vi "Desonatter Torque data read.vi"() -> (3 "Result":bool, 10 "Parameter":u8, 11 "Channel":i32)   [LabVIEW 2015]
uses:
  Galobal variable_TI.vi
  Project Setup/Globle Variable/GR_Servo.vi
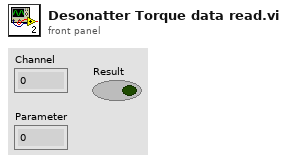
[diagram p1: front panel]
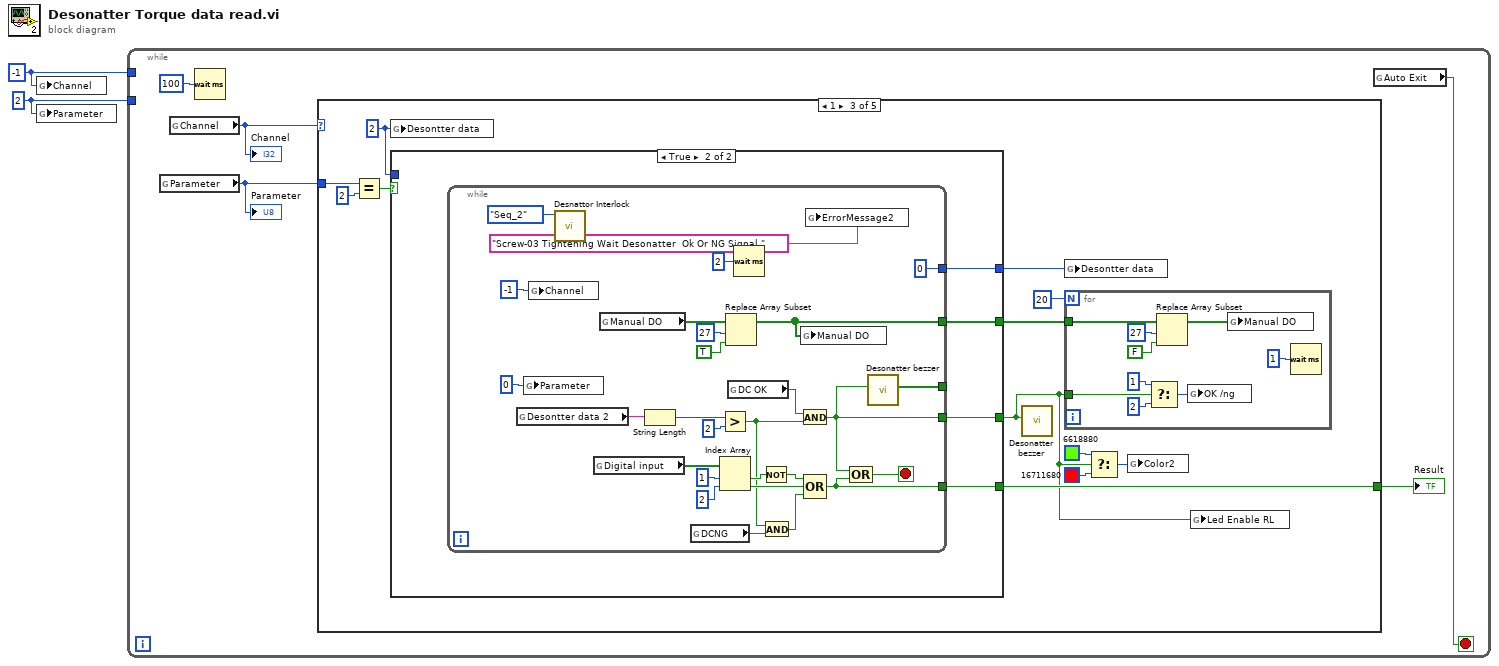
[diagram p0: block diagram]
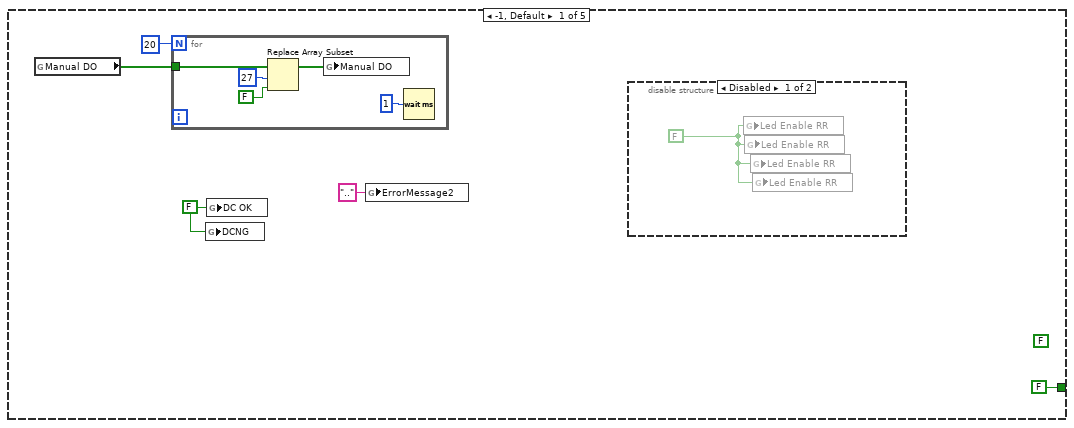
[diagram p2: hidden frame]
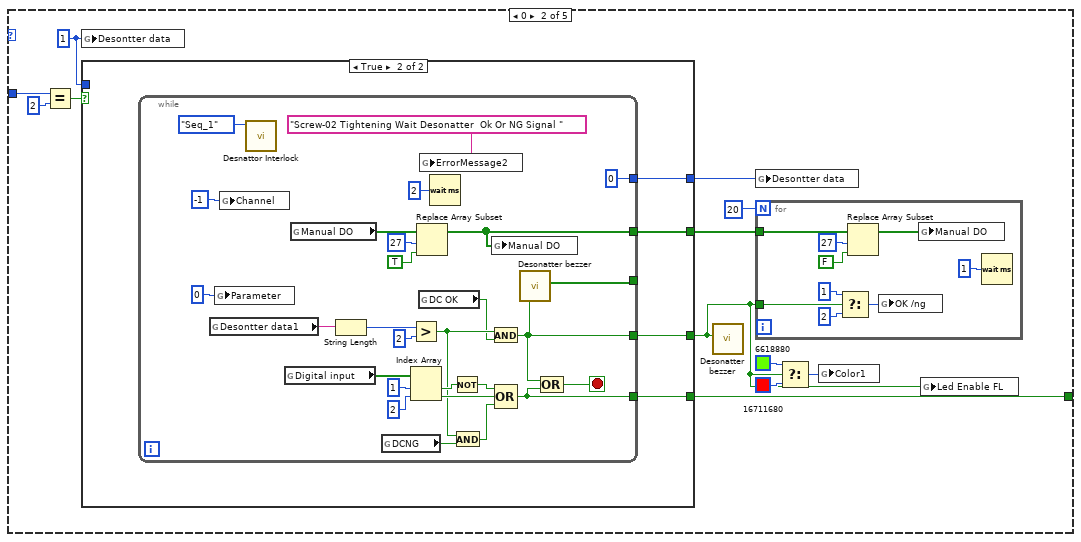
[diagram p4: hidden frame]
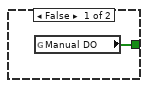
[diagram p5: hidden frame]
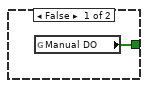
[diagram p6: hidden frame]
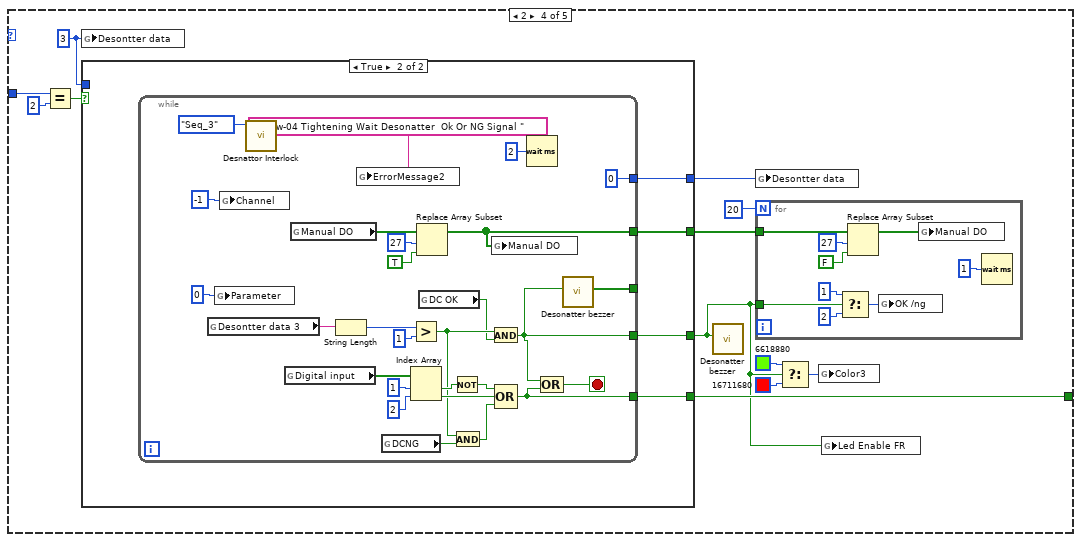
[diagram p7: hidden frame]
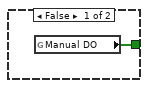
[diagram p8: hidden frame]
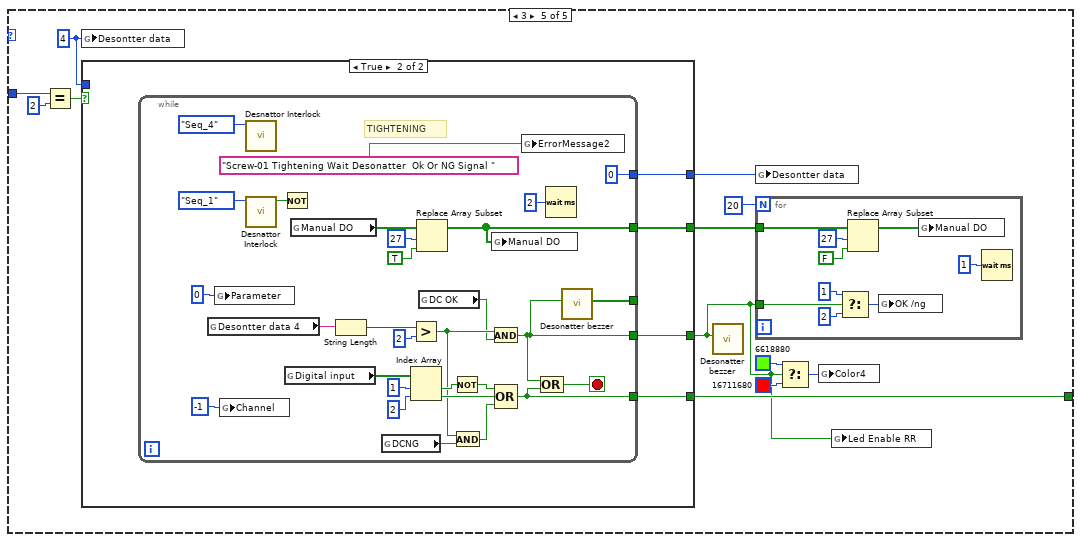
[diagram p9: hidden frame]
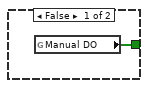
[diagram p10: hidden frame]
diagram:
  w1 = u8 2 ("Parameter")
  w2 = -1 ("Channel")
  n1 = global write "Galobal variable_TI.vi" "Channel"(w2) -> ()
  n2 = global write "Galobal variable_TI.vi" "Parameter"(w1) -> ()
  n3 = while {
    tunnel: w2 -> [_]
    tunnel: w1 -> [_]
    stop <- w6 stop-if-true
    n4 = global read "Galobal variable_TI.vi" "Parameter"() -> (w4:u8)
    "Parameter" <- w4
    n5 = global read "Galobal variable_TI.vi" "Channel"() -> (w5:i32)
    "Channel" <- w5
    n6 = Wait (ms)(milliseconds to wait=u32 100) -> ()  [unwired: 1 out]
    n7 = case shown="1" w5 {
      tunnel: w4 -> [_ w30 w83 w134 w187]
      tunnel: [FALSE w27 w82 w133 w186] -> w7
      frame -1, Default {
        (unwired) FALSE
        w8 = FALSE ("DC OK")
        n8 = global read "Galobal variable_TI.vi" "Manual DO"() -> (w11:bool[])
        n9 = for {
          N: 20 -> [_]
          tunnel: w11 -> [w18]
          n10 = Replace Array Subset(array=w18, new element=FALSE ("new element/subarray"), index=27) -> (w17:bool[])
          n11 = global write "Galobal variable_TI.vi" "Manual DO"(w17) -> ()
          n12 = Wait (ms)(milliseconds to wait=u32 1) -> ()  [unwired: 1 out]
        }
        n13 = global write "Galobal variable_TI.vi" "DCNG"(w8) -> ()
        n14 = global write "Galobal variable_TI.vi" "DC OK"(w8) -> ()
        n15 = global write "GR_Servo.vi" "ErrorMessage2"(".." ("ErrorMessage2")) -> ()
        n16 = disable-structure shown="Disabled" {
          frame Disabled {
            w13 = FALSE
            n17 = global write "Galobal variable_TI.vi" "Led Enable RR"(w13) -> ()
            n18 = global write "Galobal variable_TI.vi" "Led Enable RR"(w13) -> ()
            n19 = global write "Galobal variable_TI.vi" "Led Enable RR"(w13) -> ()
            n20 = global write "Galobal variable_TI.vi" "Led Enable RR"(w13) -> ()
          }
          frame Enabled {
          }
        }
      }
      frame 0 {
        w22 = 1 ("Desontter data")
        n21 = Equal?(x=w30, y=u8 2) -> (x = y?=w28:bool)
        n22 = global write "Galobal variable_TI.vi" "Desontter data"(w22) -> ()
        n23 = case shown="True" w28 {
          tunnel: [_ w44] -> w27
          tunnel: [_ w43] -> w26
          tunnel: [_ w42] -> w19
          tunnel: w22 -> [_ _]
          tunnel: [w40 w41] -> w21
          frame False {
            n24 = global read "Galobal variable_TI.vi" "Manual DO"() -> (w40:bool[])
          }
          frame True {
            n25 = while {
              tunnel: [w63] -> w44
              tunnel: [0 ("y")] -> w43
              tunnel: [w45] -> w42
              tunnel: [w53] -> w41
              tunnel: [w48] -> _
              stop <- w62 stop-if-true
              n26 = global read "Galobal variable_TI.vi" "Desontter data1"() -> (w66:string)
              n27 = global write "Galobal variable_TI.vi" "Parameter"(u8 0 ("Parameter")) -> ()
              n28 = global write "Galobal variable_TI.vi" "Channel"(-1 ("Channel")) -> ()
              n29 = call "Desnattor Interlock.vi"("Seq1"=enum16{"Seq_1", "Seq_2", "Seq_3", "Seq_4"}."Seq_1") -> ()  [unwired: 10 in, 1 out]
              n30 = global read "Galobal variable_TI.vi" "Digital input"() -> (w60:bool[])
              n31 = global read "Galobal variable_TI.vi" "Manual DO"() -> (w55:bool[])
              n32 = String Length(string=w66) -> (length=w65:i32)
              n33 = global read "Galobal variable_TI.vi" "DCNG"() -> (w58:bool)
              n34 = Greater?(x=w65, y=2) -> (0:w59:bool)
              n35 = Index Array(array=w60, index #1=1 ("index"), index #2=2 ("index")) -> (element #1=w69:bool, element #2=w67:bool)
              n36 = Replace Array Subset(array=w55, new element=TRUE ("new element/subarray"), index=27) -> (w53:bool[])
              n37 = global read "Galobal variable_TI.vi" "DC OK"() -> (w49:bool)
              n38 = global write "GR_Servo.vi" "ErrorMessage2"("Screw-02 Tightening Wait Desonatter  Ok Or NG Signal ") -> ()
              n39 = Wait (ms)(milliseconds to wait=u32 2) -> ()  [unwired: 1 out]
              n40 = Not(x=w69) -> (.not. x?=w68:bool)
              n41 = And(x=w59, y=w58) -> (x .and. y?=w57:bool)
              n42 = And(x=w59, y=w49) -> (x .and. y?=w45:bool)
              n43 = global write "Galobal variable_TI.vi" "Manual DO"(w53) -> ()
              n44 = Compound Arithmetic op=OR(w68, w67, w57) -> (w63:bool)
              n45 = call "Desonatter bezzer.vi"("OK"=w45) -> ("Array"=w48:bool[])  [unwired: 10 in]
              n46 = Compound Arithmetic op=OR(w45, w63) -> (w62:bool)
            }
          }
        }
        n47 = call "Desonatter bezzer.vi"("OK"=w19) -> ()  [unwired: 10 in, 1 out]
        n48 = global write "Galobal variable_TI.vi" "Desontter data"(w26) -> ()
        n49 = for {
          N: 20 -> [_]
          tunnel: w21 -> [w39]
          tunnel: w19 -> [w31]
          n50 = Select(t=1, s=w31, f=2) -> (s? t:f=w34:i32)
          n51 = Replace Array Subset(array=w39, new element=FALSE ("new element/subarray"), index=27) -> (w38:bool[])
          n52 = global write "Galobal variable_TI.vi" "OK /ng"(w34) -> ()
          n53 = global write "Galobal variable_TI.vi" "Manual DO"(w38) -> ()
          n54 = Wait (ms)(milliseconds to wait=u32 1) -> ()  [unwired: 1 out]
        }
        n55 = Select(t=u32 6618880 ("Color Box"), s=w19, f=u32 16711680 ("Color Box")) -> (s? t:f=w23:u32)
        n56 = global write "Galobal variable_TI.vi" "Color1"(w23) -> ()
        n57 = global write "Galobal variable_TI.vi" "Led Enable FL"(w19) -> ()
      }
      frame 1 {
        w75 = 2 ("Desontter data")
        n58 = Equal?(x=w83, y=u8 2) -> (x = y?=w80:bool)
        n59 = global write "Galobal variable_TI.vi" "Desontter data"(w75) -> ()
        n60 = case shown="True" w80 {
          tunnel: [_ w97] -> w82
          tunnel: [_ w96] -> w79
          tunnel: [_ w95] -> w72
          tunnel: w75 -> [_ _]
          tunnel: [w93 w94] -> w73
          frame False {
            n61 = global read "Galobal variable_TI.vi" "Manual DO"() -> (w93:bool[])
          }
          frame True {
            n62 = while {
              tunnel: [w115] -> w97
              tunnel: [0 ("y")] -> w96
              tunnel: [w98] -> w95
              tunnel: [w105] -> w94
              tunnel: [w101] -> _
              stop <- w114 stop-if-true
              n63 = global read "Galobal variable_TI.vi" "Desontter data 2"() -> (w118:string)
              n64 = global write "Galobal variable_TI.vi" "Parameter"(u8 0 ("Parameter")) -> ()
              n65 = global write "Galobal variable_TI.vi" "Channel"(-1 ("Channel")) -> ()
              n66 = call "Desnattor Interlock.vi"("Seq1"=enum16{"Seq_1", "Seq_2", "Seq_3", "Seq_4"}."Seq_2") -> ()  [unwired: 10 in, 1 out]
              n67 = global read "Galobal variable_TI.vi" "Digital input"() -> (w124:bool[])
              n68 = global read "Galobal variable_TI.vi" "Manual DO"() -> (w108:bool[])
              n69 = String Length(string=w118) -> (length=w117:i32)
              n70 = global read "Galobal variable_TI.vi" "DCNG"() -> (w111:bool)
              n71 = Greater?(x=w117, y=2) -> (0:w112:bool)
              n72 = Index Array(array=w124, index #1=1 ("index"), index #2=2 ("index")) -> (element #1=w121:bool, element #2=w119:bool)
              n73 = Replace Array Subset(array=w108, new element=TRUE ("new element/subarray"), index=27) -> (w105:bool[])
              n74 = global read "Galobal variable_TI.vi" "DC OK"() -> (w102:bool)
              n75 = Wait (ms)(milliseconds to wait=u32 2) -> ()  [unwired: 1 out]
              n76 = Not(x=w121) -> (.not. x?=w120:bool)
              n77 = And(x=w112, y=w111) -> (x .and. y?=w110:bool)
              n78 = And(x=w102, y=w112) -> (x .and. y?=w98:bool)
              n79 = global write "Galobal variable_TI.vi" "Manual DO"(w105) -> ()
              n80 = Compound Arithmetic op=OR(w120, w119, w110) -> (w115:bool)
              n81 = global write "GR_Servo.vi" "ErrorMessage2"("Screw-03 Tightening Wait Desonatter  Ok Or NG Signal ") -> ()
              n82 = Compound Arithmetic op=OR(w98, w115) -> (w114:bool)
              n83 = call "Desonatter bezzer.vi"("OK"=w98) -> ("Array"=w101:bool[])  [unwired: 10 in]
            }
          }
        }
        n84 = call "Desonatter bezzer.vi"("OK"=w72) -> ()  [unwired: 10 in, 1 out]
        n85 = global write "Galobal variable_TI.vi" "Desontter data"(w79) -> ()
        n86 = for {
          N: 20 -> [_]
          tunnel: w73 -> [w92]
          tunnel: w72 -> [w87]
          n87 = Select(t=1, s=w87, f=2) -> (s? t:f=w86:i32)
          n88 = Replace Array Subset(array=w92, new element=FALSE ("new element/subarray"), index=27) -> (w91:bool[])
          n89 = global write "Galobal variable_TI.vi" "OK /ng"(w86) -> ()
          n90 = global write "Galobal variable_TI.vi" "Manual DO"(w91) -> ()
          n91 = Wait (ms)(milliseconds to wait=u32 1) -> ()  [unwired: 1 out]
        }
        n92 = Select(t=u32 6618880 ("Color Box"), s=w72, f=u32 16711680 ("Color Box")) -> (s? t:f=w78:u32)
        n93 = global write "Galobal variable_TI.vi" "Color2"(w78) -> ()
        n94 = global write "Galobal variable_TI.vi" "Led Enable RL"(w72) -> ()
      }
      frame 2 {
        w128 = 3 ("Desontter data")
        n95 = Equal?(x=w134, y=u8 2) -> (x = y?=w135:bool)
        n96 = global write "Galobal variable_TI.vi" "Desontter data"(w128) -> ()
        n97 = case shown="True" w135 {
          tunnel: [_ w150] -> w133
          tunnel: [_ w149] -> w132
          tunnel: [_ w148] -> w125
          tunnel: w128 -> [_ _]
          tunnel: [w146 w147] -> w126
          frame False {
            n98 = global read "Galobal variable_TI.vi" "Manual DO"() -> (w146:bool[])
          }
          frame True {
            n99 = while {
              tunnel: [w168] -> w150
              tunnel: [0 ("y")] -> w149
              tunnel: [w151] -> w148
              tunnel: [w158] -> w147
              tunnel: [w154] -> _
              stop <- w167 stop-if-true
              n100 = global read "Galobal variable_TI.vi" "Desontter data 3"() -> (w171:string)
              n101 = global write "Galobal variable_TI.vi" "Parameter"(u8 0 ("Parameter")) -> ()
              n102 = global write "Galobal variable_TI.vi" "Channel"(-1 ("Channel")) -> ()
              n103 = call "Desnattor Interlock.vi"("Seq1"=enum16{"Seq_1", "Seq_2", "Seq_3", "Seq_4"}."Seq_3") -> ()  [unwired: 10 in, 1 out]
              n104 = global read "Galobal variable_TI.vi" "Digital input"() -> (w177:bool[])
              n105 = global read "Galobal variable_TI.vi" "Manual DO"() -> (w161:bool[])
              n106 = String Length(string=w171) -> (length=w170:i32)
              n107 = global write "GR_Servo.vi" "ErrorMessage2"("Screw-04 Tightening Wait Desonatter  Ok Or NG Signal ") -> ()
              n108 = global read "Galobal variable_TI.vi" "DCNG"() -> (w163:bool)
              n109 = Greater?(x=w170, y=1) -> (0:w165:bool)
              n110 = Index Array(array=w177, index #1=1 ("index"), index #2=2 ("index")) -> (element #1=w174:bool, element #2=w172:bool)
              n111 = Replace Array Subset(array=w161, new element=TRUE ("new element/subarray"), index=27) -> (w158:bool[])
              n112 = global read "Galobal variable_TI.vi" "DC OK"() -> (w155:bool)
              n113 = Not(x=w174) -> (.not. x?=w173:bool)
              n114 = And(x=w165, y=w163) -> (x .and. y?=w164:bool)
              n115 = And(x=w165, y=w155) -> (x .and. y?=w151:bool)
              n116 = global write "Galobal variable_TI.vi" "Manual DO"(w158) -> ()
              n117 = Compound Arithmetic op=OR(w173, w172, w164) -> (w168:bool)
              n118 = Wait (ms)(milliseconds to wait=u32 2) -> ()  [unwired: 1 out]
              n119 = Compound Arithmetic op=OR(w151, w168) -> (w167:bool)
              n120 = call "Desonatter bezzer.vi"("OK"=w151) -> ("Array"=w154:bool[])  [unwired: 10 in]
            }
          }
        }
        n121 = call "Desonatter bezzer.vi"("OK"=w125) -> ()  [unwired: 10 in, 1 out]
        n122 = global write "Galobal variable_TI.vi" "Desontter data"(w132) -> ()
        n123 = for {
          N: 20 -> [_]
          tunnel: w126 -> [w145]
          tunnel: w125 -> [w137]
          n124 = Select(t=1, s=w137, f=2) -> (s? t:f=w140:i32)
          n125 = Replace Array Subset(array=w145, new element=FALSE ("new element/subarray"), index=27) -> (w144:bool[])
          n126 = global write "Galobal variable_TI.vi" "OK /ng"(w140) -> ()
          n127 = global write "Galobal variable_TI.vi" "Manual DO"(w144) -> ()
          n128 = Wait (ms)(milliseconds to wait=u32 1) -> ()  [unwired: 1 out]
        }
        n129 = Select(t=u32 6618880 ("Color Box"), s=w125, f=u32 16711680 ("Color Box")) -> (s? t:f=w131:u32)
        n130 = global write "Galobal variable_TI.vi" "Color3"(w131) -> ()
        n131 = global write "Galobal variable_TI.vi" "Led Enable FR"(w125) -> ()
      }
      frame 3 {
        w181 = 4 ("Desontter data")
        n132 = Equal?(x=w187, y=u8 2) -> (x = y?=w188:bool)
        n133 = global write "Galobal variable_TI.vi" "Desontter data"(w181) -> ()
        n134 = case shown="True" w188 {
          tunnel: [_ w203] -> w186
          tunnel: [_ w202] -> w185
          tunnel: [_ w201] -> w178
          tunnel: w181 -> [_ _]
          tunnel: [w199 w200] -> w179
          frame False {
            n135 = global read "Galobal variable_TI.vi" "Manual DO"() -> (w199:bool[])
          }
          frame True {
            n136 = while {
              tunnel: [w223] -> w203
              tunnel: [0 ("Desontter data")] -> w202
              tunnel: [w204] -> w201
              tunnel: [w210] -> w200
              tunnel: [w206] -> _
              stop <- w222 stop-if-true
              # "TIGHTENING"
              n137 = global read "Galobal variable_TI.vi" "Desontter data 4"() -> (w226:string)
              n138 = global write "Galobal variable_TI.vi" "Parameter"(u8 0 ("Parameter")) -> ()
              n139 = global write "Galobal variable_TI.vi" "Channel"(-1 ("Channel")) -> ()
              n140 = call "Desnattor Interlock.vi"("Seq1"=enum16{"Seq_1", "Seq_2", "Seq_3", "Seq_4"}."Seq_4") -> ()  [unwired: 10 in, 1 out]
              n141 = call "Desnattor Interlock.vi"("Seq1"=enum16{"Seq_1", "Seq_2", "Seq_3", "Seq_4"}."Seq_1") -> ("Ready"=w215:bool)  [unwired: 10 in]
              n142 = Not(x=w215) -> ()  [unwired: 1 out]
              n143 = global read "Galobal variable_TI.vi" "Digital input"() -> (w232:bool[])
              n144 = global read "Galobal variable_TI.vi" "Manual DO"() -> (w213:bool[])
              n145 = String Length(string=w226) -> (length=w225:i32)
              n146 = global read "Galobal variable_TI.vi" "DCNG"() -> (w219:bool)
              n147 = Greater?(x=w225, y=2) -> (0:w218:bool)
              n148 = Index Array(array=w232, index #1=1 ("index"), index #2=2 ("index")) -> (element #1=w229:bool, element #2=w227:bool)
              n149 = Replace Array Subset(array=w213, new element=TRUE ("new element/subarray"), index=27) -> (w210:bool[])
              n150 = global read "Galobal variable_TI.vi" "DC OK"() -> (w207:bool)
              n151 = Not(x=w229) -> (.not. x?=w228:bool)
              n152 = And(x=w218, y=w219) -> (x .and. y?=w217:bool)
              n153 = And(x=w218, y=w207) -> (x .and. y?=w204:bool)
              n154 = global write "Galobal variable_TI.vi" "Manual DO"(w210) -> ()
              n155 = Compound Arithmetic op=OR(w228, w227, w217) -> (w223:bool)
              n156 = global write "GR_Servo.vi" "ErrorMessage2"("Screw-01 Tightening Wait Desonatter  Ok Or NG Signal ") -> ()
              n157 = Compound Arithmetic op=OR(w204, w223) -> (w222:bool)
              n158 = Wait (ms)(milliseconds to wait=u32 2) -> ()  [unwired: 1 out]
              n159 = call "Desonatter bezzer.vi"("OK"=w204) -> ("Array"=w206:bool[])  [unwired: 10 in]
            }
          }
        }
        n160 = call "Desonatter bezzer.vi"("OK"=w178) -> ()  [unwired: 10 in, 1 out]
        n161 = global write "Galobal variable_TI.vi" "Desontter data"(w185) -> ()
        n162 = for {
          N: 20 -> [_]
          tunnel: w179 -> [w198]
          tunnel: w178 -> [w190]
          n163 = Select(t=1, s=w190, f=2) -> (s? t:f=w193:i32)
          n164 = Replace Array Subset(array=w198, new element=FALSE ("new element/subarray"), index=27) -> (w197:bool[])
          n165 = global write "Galobal variable_TI.vi" "OK /ng"(w193) -> ()
          n166 = global write "Galobal variable_TI.vi" "Manual DO"(w197) -> ()
          n167 = Wait (ms)(milliseconds to wait=u32 1) -> ()  [unwired: 1 out]
        }
        n168 = Select(t=u32 6618880 ("Color Box"), s=w178, f=u32 16711680 ("Color Box")) -> (s? t:f=w184:u32)
        n169 = global write "Galobal variable_TI.vi" "Color4"(w184) -> ()
        n170 = global write "Galobal variable_TI.vi" "Led Enable RR"(w178) -> ()
      }
    }
    "Result" <- w7
    n171 = global read "Galobal variable_TI.vi" "Auto Exit"() -> (w6:bool)
  }
